vi "get Pmu Configuration Labview.vi"(7 "pmuIndex":i32, 9 "pseudoPdcId":i32, 10 "stationName":string, 11 "pmuconf":T1) -> (1 "function return":i32, 2 "stationName out":string, 3 "pmuconf out":T1)   [LabVIEW 2018, in "S3DK.lvlib" / "C37118-DLL.lvlib" / "StrongridDLL.lvlib"]
doc: "STRONGRIDIEEEC37118DLL_API int __cdecl getPmuConfigurationLabview(noArraysPmuConfig* pmuconf, char* stationName, int32_t pseudoPdcId, int32_t pmuIndex);"
uses:
  StrongridDLL.lvlib
  <vilib>/builds/S3DK Compiler/My Packed Library/StrongridDLL.dll
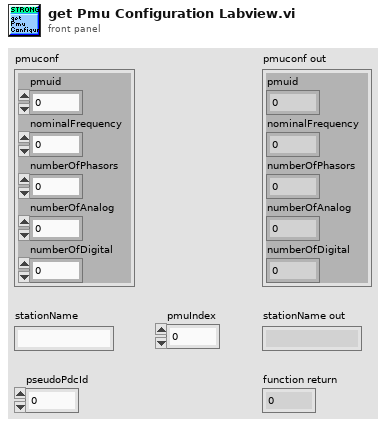
[diagram p1: front panel]
types:
  T1 = cluster{"pmuid":i32, "nominalFrequency":sgl, "numberOfPhasors":i32, "numberOfAnalog":i32, "numberOfDigital":i32}
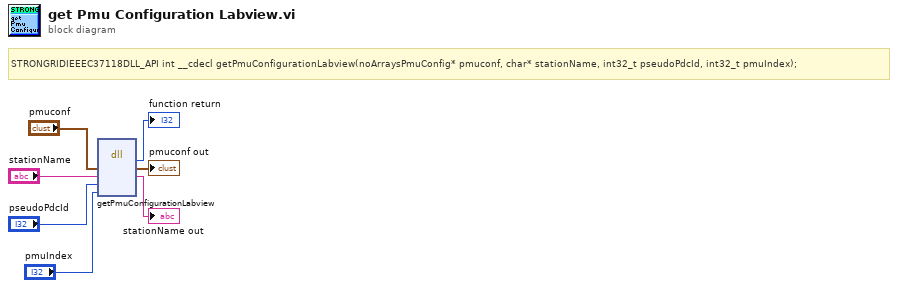
[diagram p0: block diagram]
diagram:
  # "STRONGRIDIEEEC37118DLL_API int __cdecl getPmuConfigurationLabview(noArraysPmuConfig* pmuconf, char* stationName, int32_t pseudoPdcId, int32_t pmuIndex);"
  n1 = dll-call lib="C:/Program Files/National Instruments/LabVIEW 2018/vi.lib/builds/S3DK Compiler/My Packed Library/StrongridDLL.*" fn="getPmuConfigurationLabview"("pmuconf"="pmuconf", "stationName"="stationName", "pseudoPdcId"="pseudoPdcId", "pmuIndex"="pmuIndex") -> (→"function return":i32, "pmuconf"=→"pmuconf out":T1, "stationName"=→"stationName out":string)  [unwired: 5 in, 2 out]
